vi "FrontPanel.vi"(8 "error in (no error)":errorcluster) -> (0 "error out":errorcluster)   [LabVIEW 2021]
uses:
  <vilib>/Native 3D Graph/xcontrol/3DPC_SurfacePlot.xctl
  QueueEnum.ctl
  ToViewQueueData.ctl
  ViewUpdateEnum.ctl
  ToControllerQueueCluster.ctl
  ToControllerEnum.ctl
panel:
  in  "Slide":dbl(slide) scale=0.0..100.0
  in  "See data from log file":bool
  in  "saving logs":bool
  in  "Log file":path
  in  "stop":bool
  in  "Send":bool
  in  "Message To Send":string
  out "3D Graph":refnum<class "Base Datatype.lvclass">[](xcontrol)
  out "Connected?":bool
  in  "Disconnect":bool
  in  "Connect":bool
  in  "Remote Port Number":u16
  in  "Server IP":string
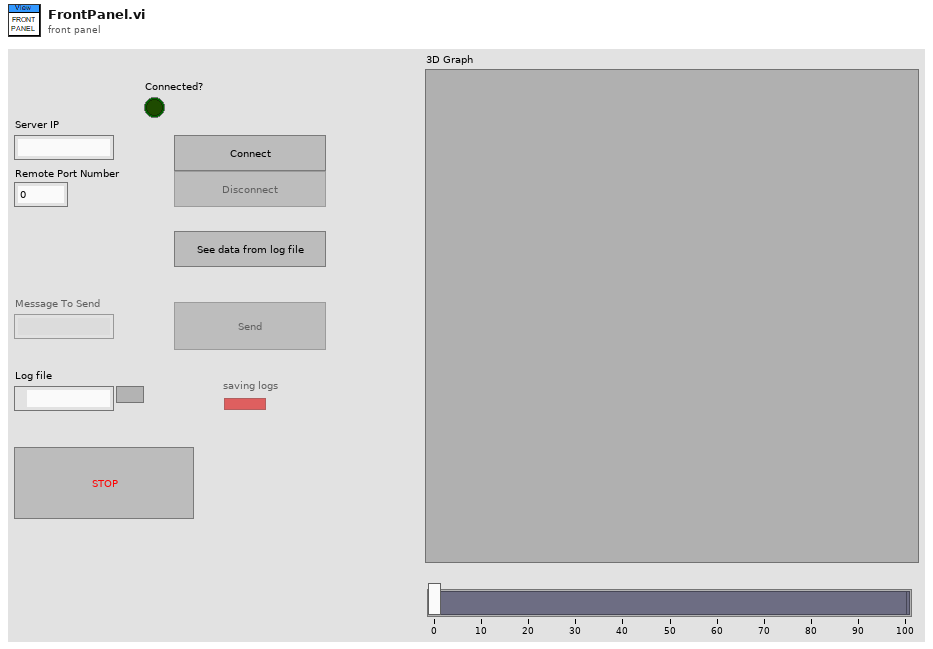
[diagram p1: front panel]
types:
  T1 = typedef "ToViewQueueData.ctl" = cluster{"DataToUpdate":T2, "ConnectionStatus":bool, "GraphData":dbl[][], "Message":string}
  T2 = typedef "ViewUpdateEnum.ctl" = enum16{"Init", "OneButtonMessage", "Exit", "UpdateButtonsEnabled", "UpdateGraph", "UpdateConnectionStatus"}
  T3 = enum32{"Bad", "Idle", "Run top level", "Running"}
  T4 = typedef "QueueEnum.ctl" = enum16{"Obtain Queue", "Get Queue Ref", "Flush Queue", "Release Queue"}
  T5 = typedef "ToControllerEnum.ctl" = enum16{"Info_Disconnected", "Info_Connected", "Exit", "Disconnect", "Connect", "SendMessage", "Slide", "ShowDataFromLog", "Start_Saving_Logs", "Stop_Saving_Logs"}
  T6 = typedef "ToControllerQueueCluster.ctl" = cluster{"Message":T5, "Remote IP":string, "Remote Port":u16, "Data":string}
  T7 = enum8{"Enabled", "Disabled", "Disabled and Grayed Out"}
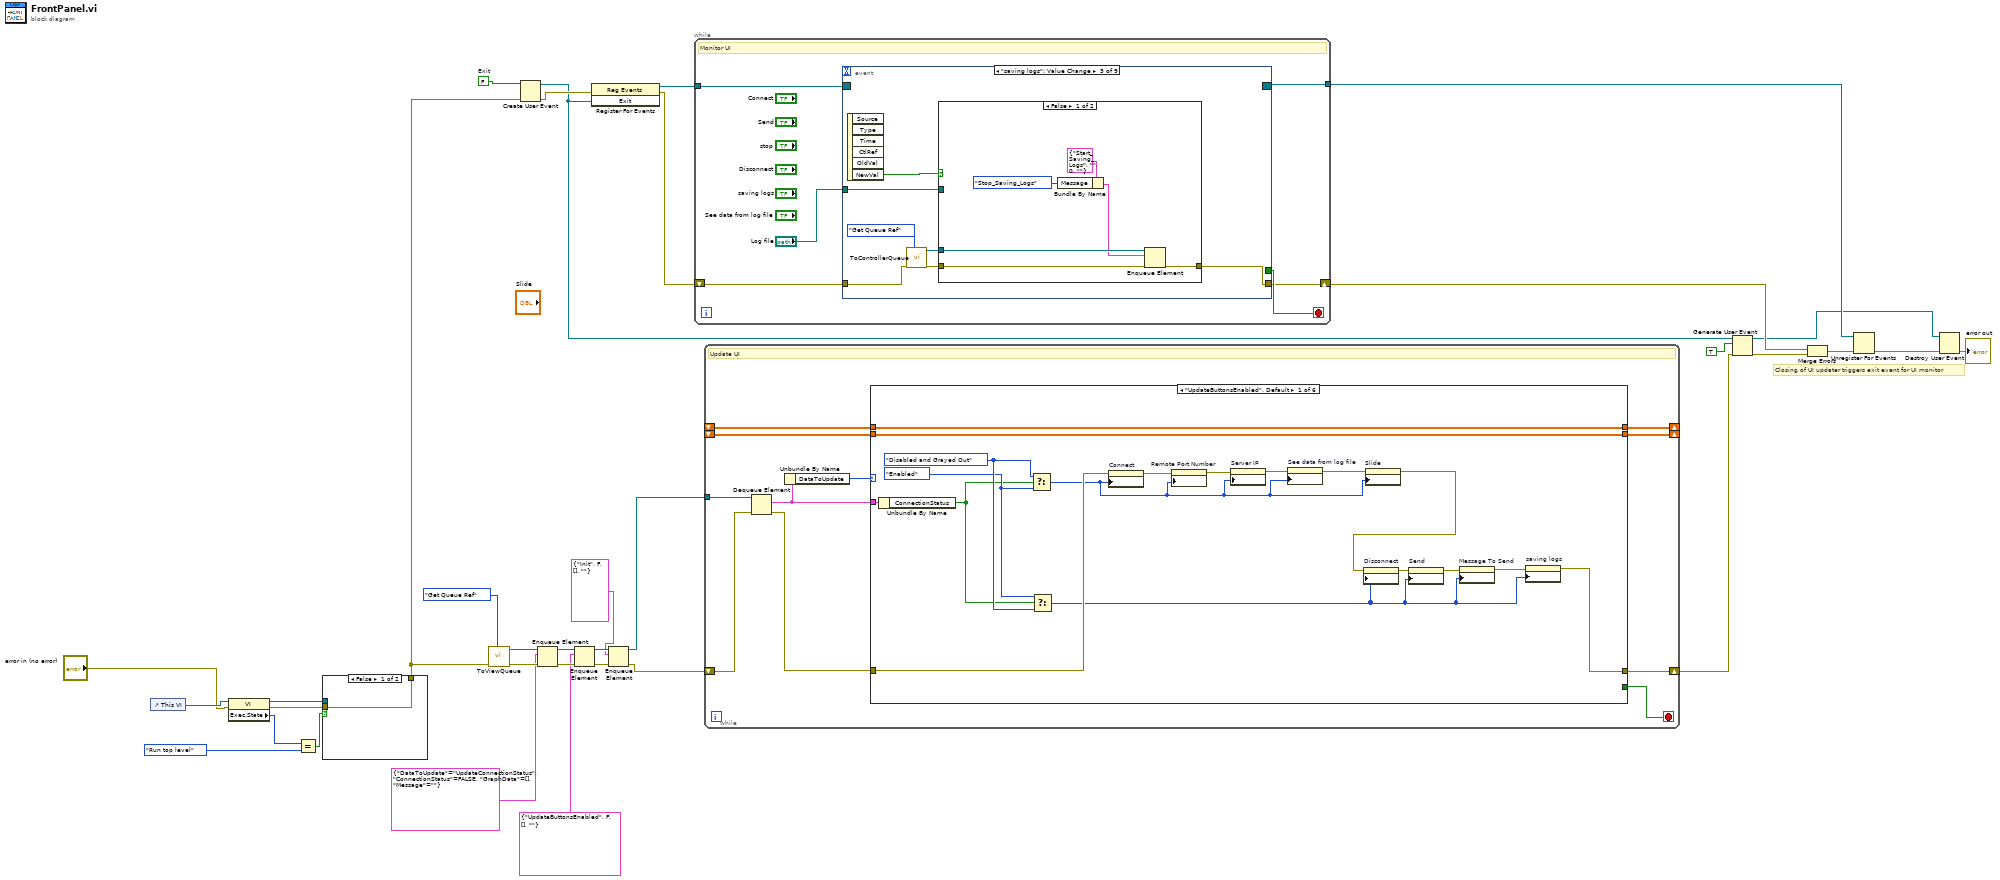
[diagram p0: block diagram]
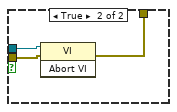
[diagram p2: hidden frame]
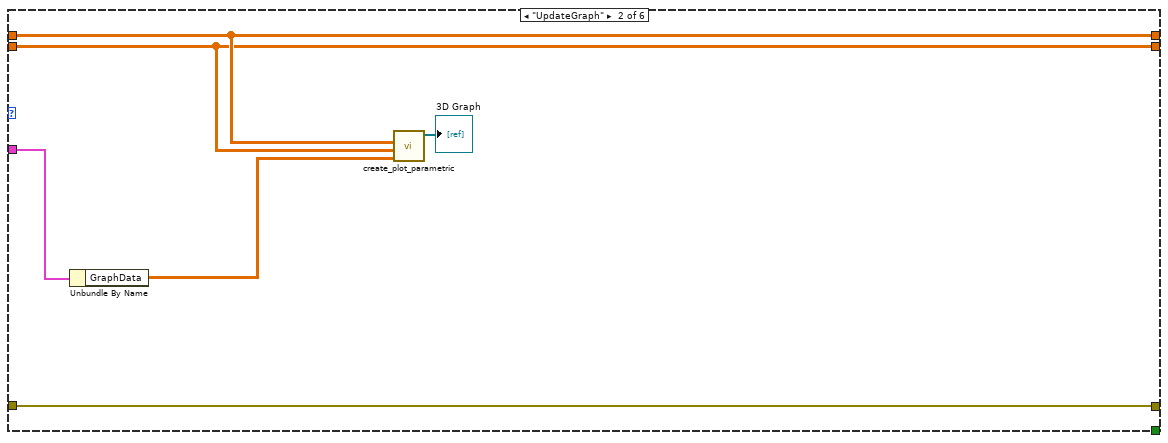
[diagram p3: hidden frame]
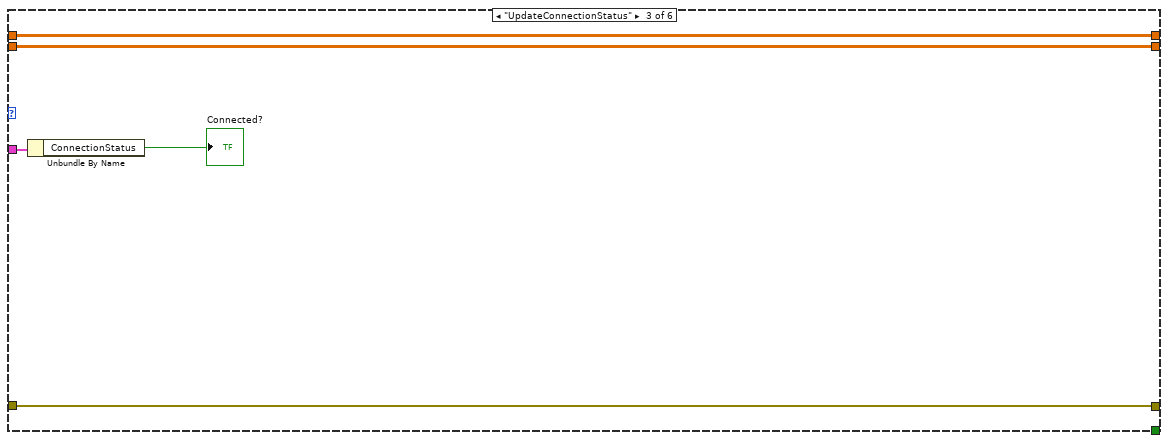
[diagram p4: hidden frame]
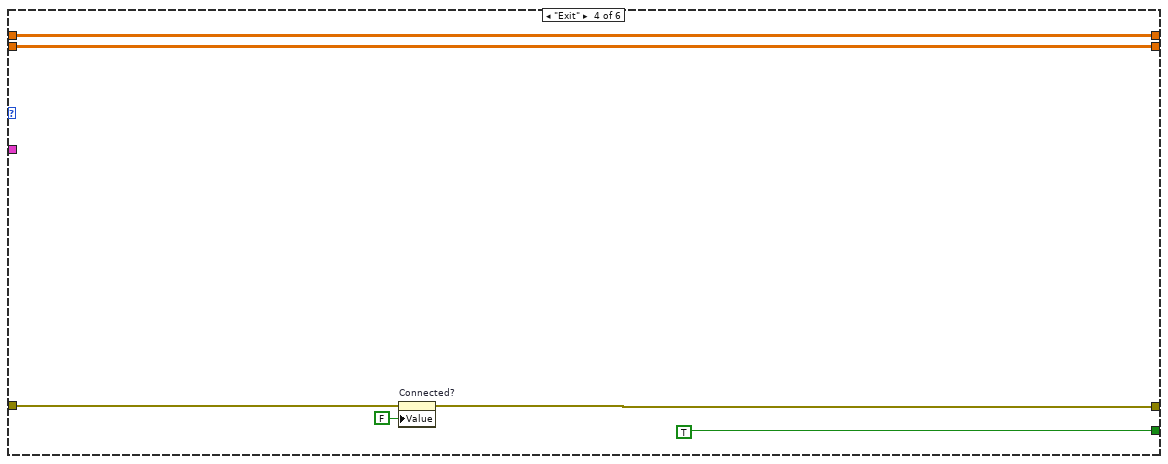
[diagram p5: hidden frame]
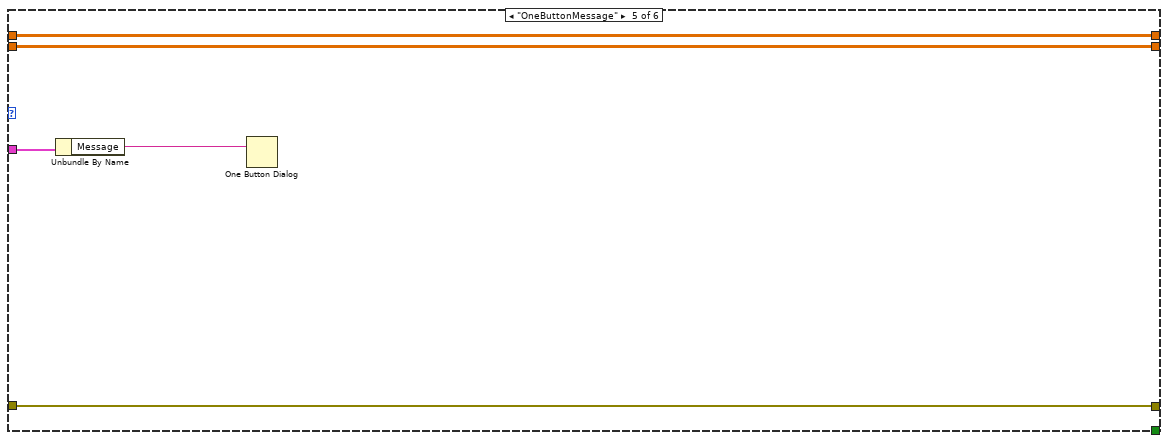
[diagram p6: hidden frame]
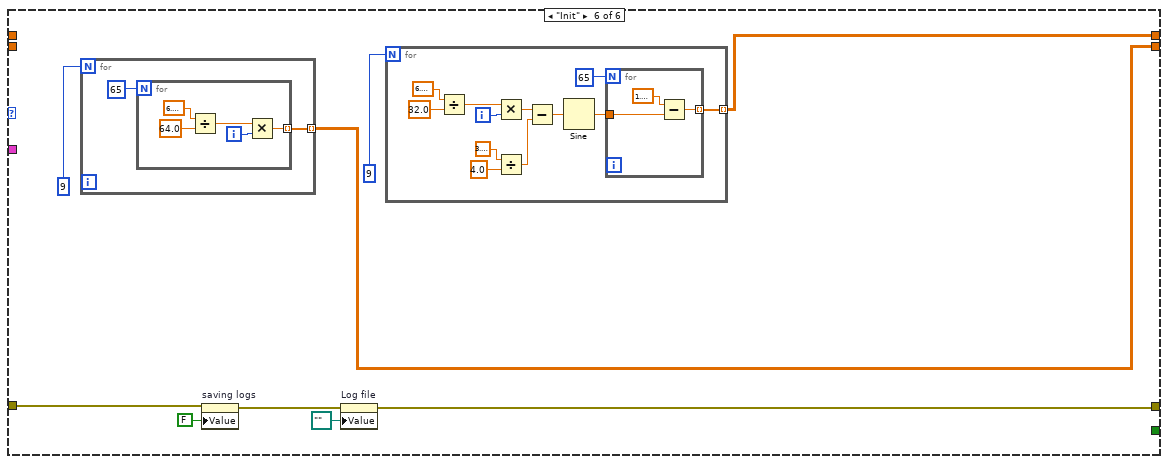
[diagram p7: hidden frame]
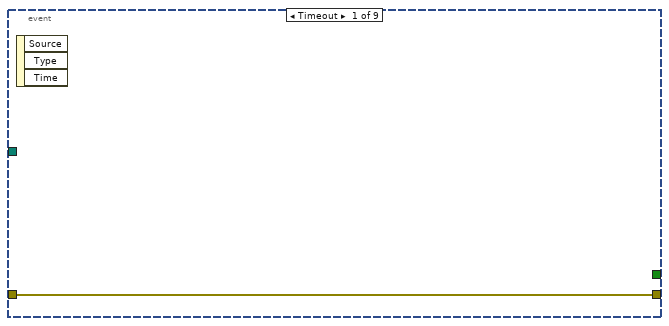
[diagram p8: hidden frame]
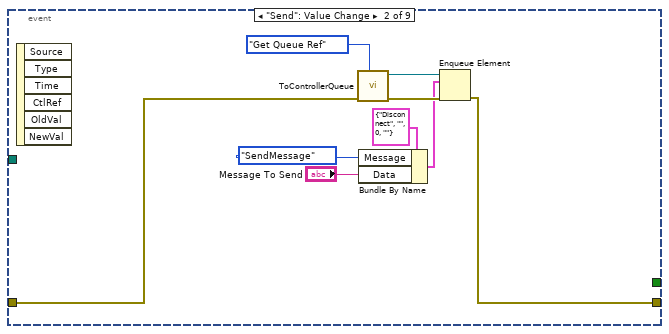
[diagram p9: hidden frame]
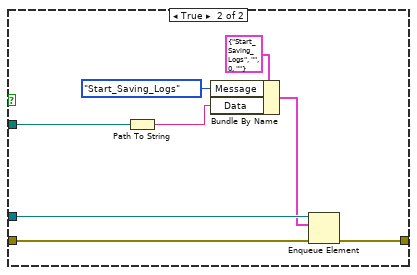
[diagram p10: hidden frame]
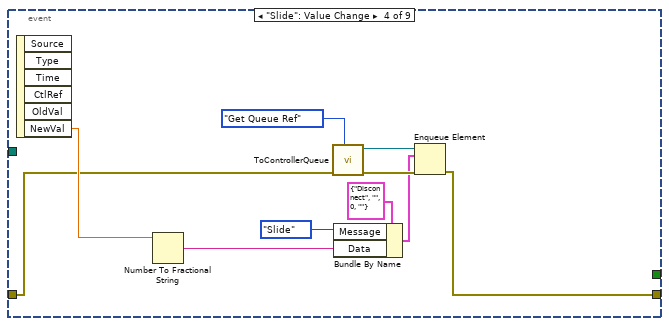
[diagram p11: hidden frame]
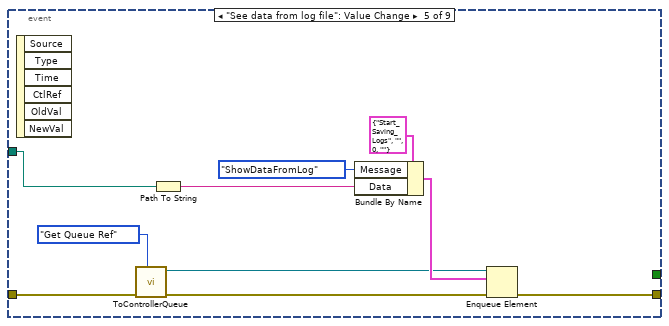
[diagram p12: hidden frame]
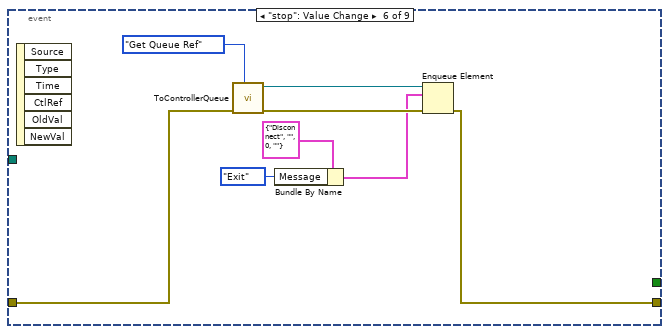
[diagram p13: hidden frame]
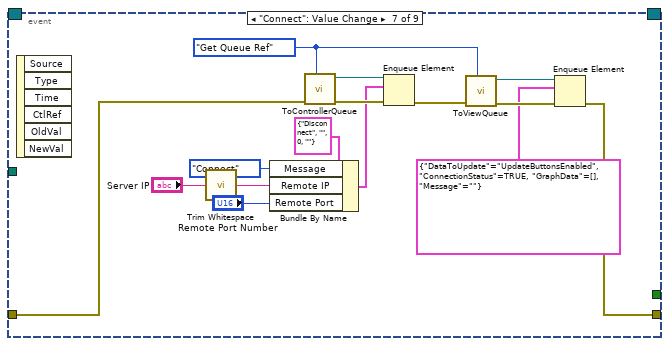
[diagram p14: hidden frame]
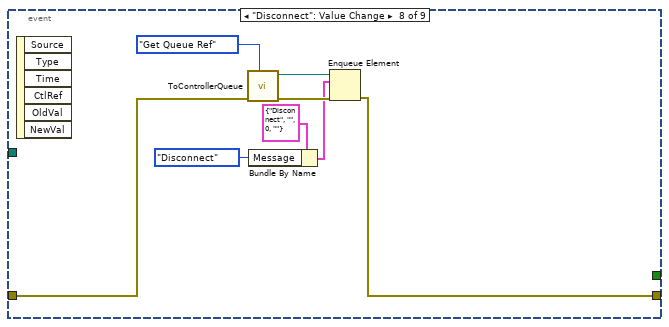
[diagram p15: hidden frame]
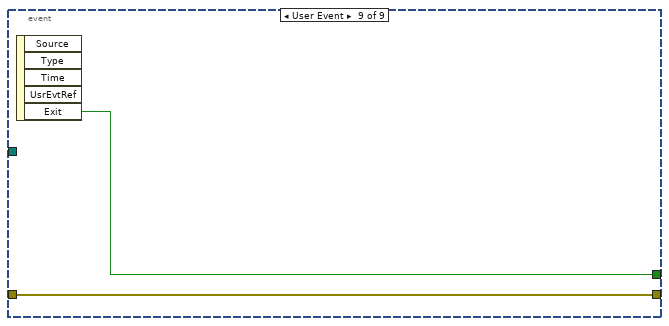
[diagram p16: hidden frame]
diagram:
  w33 = FALSE  # Exit
  # "Closing of UI updater triggers exit event for UI monitor"
  n1 = control-ref of="This VI"() -> (w17:refnum<vi>)
  n2 = property class="VI"(reference=w17, error in="error in (no error)") -> (reference out=w13:refnum<vi>, error out=w14:errorcluster, "Exec.State"=w15:T3)
  n3 = Equal?(x=w15, y=T3."Run top level" ("Execution:State")) -> (x = y?=w11:bool)
  n4 = case shown="False" w11 {
    tunnel: w14 -> [w35 w38]
    tunnel: w13 -> [_ w37]
    tunnel: [w35 w36] -> w21
    frame False {
    }
    frame True {
      n5 = invoke class="VI" method="Abort VI"(reference=w37, error in=w38) -> (error out=w36:errorcluster)  [unwired: 1 in, 2 out]
    }
  }
  n6 = call "ToViewQueue.vi"("Enum"=QueueEnum."Get Queue Ref", "error in (no error)"=w21) -> ("error out"=w9:errorcluster, "queue out"=w19:refnum<queue>)  [unwired: 8 in]
  n7 = Create User Event(user event datatype=w33, error in=w21) -> (user event=w23:refnum<user-event>, error out=w34:errorcluster)
  n8 = Enqueue Element(queue=w19, element=T1 {"DataToUpdate"=enum."UpdateConnectionStatus", "ConnectionStatus"=FALSE, "GraphData"=[], "Message"=""}, error in (no error)=w9) -> (queue out=w10:refnum<queue>, error out=w7:errorcluster)  [unwired: 1 in, 1 out]
  n9 = Enqueue Element(queue=w10, element=T1 {"DataToUpdate"=enum."UpdateButtonsEnabled", "ConnectionStatus"=FALSE, "GraphData"=[], "Message"=""}, error in (no error)=w7) -> (queue out=w8:refnum<queue>, error out=w3:errorcluster)  [unwired: 1 in, 1 out]
  n10 = register-events(error in=w34, w23) -> (reference out=w32:refnum<event-registration>, error out=w31:errorcluster)  [unwired: 1 in]
  n11 = Enqueue Element(queue=w8, element=T1 {"DataToUpdate"=enum."Init", "ConnectionStatus"=FALSE, "GraphData"=[], "Message"=""}, error in (no error)=w3) -> (queue out=w4:refnum<queue>, error out=w2:errorcluster)  [unwired: 1 in, 1 out]
  n12 = while {
    tunnel: w32 -> [w44]
    tunnel: [w41] -> w28
    shift-right: [w40] -> w26
    shift-left: w31 -> [w43]
    stop <- w42 stop-if-true
    # "Monitor UI"
    n13 = event shown="[2] \"saving logs\": Value Change" {
      selector: w44 -> [_ _ _ _ _ _ _ _ _]
      dyn-events: [_ _ _ _ _ _ _ _ _] -> w41
      timeout: _ -> [_ _ _ _ _ _ _ _ _]
      tunnel: w43 -> [w45 w48 w58 w77 w94 w102 w116 w119 w127]
      tunnel: [_ _ _ _ _ _ _ _ w128] -> w42
      tunnel: [w45 w47 w60 w76 w88 w100 w112 w120 w127] -> w40
      tunnel: "Log file" -> [_ _ w55 _ w87 _ _ _ _]
      event Timeout {
        n14 = event-data() -> ()  [unwired: 1 in, 3 out]
      }
      event "Send": Value Change {
        n15 = event-data() -> ()  [unwired: 1 in, 6 out]
        n16 = call "ToControllerQueue.vi"("Enum"=QueueEnum."Get Queue Ref", "error in (no error)"=w48) -> ("error out"=w54:errorcluster, "queue out"=w52:refnum<queue>)  [unwired: 8 in]
        n17 = Bundle By Name(cluster=T6 {"Message"=enum."Disconnect", "Remote IP"="", "Remote Port"=0, "Data"=""} ("element"), "Message"=ToControllerEnum."SendMessage", "Data"="Message To Send") -> (w49:T6)
        n18 = Enqueue Element(queue=w52, element=w49, error in (no error)=w54) -> (error out=w47:errorcluster)  [unwired: 1 in, 2 out]
      }
      event "saving logs": Value Change {
        n19 = event-data() -> ("NewVal"=w61:bool)  [unwired: 1 in, 5 out]
        n20 = call "ToControllerQueue.vi"("Enum"=QueueEnum."Get Queue Ref", "error in (no error)"=w58) -> ("error out"=w57:errorcluster, "queue out"=w56:refnum<queue>)  [unwired: 8 in]
        n21 = case shown="False" w61 {
          tunnel: w57 -> [w66 w75]
          tunnel: [w65 w73] -> w60
          tunnel: w56 -> [w67 w74]
          tunnel: w55 -> [_ w68]
          frame False {
            n22 = Bundle By Name(cluster=T6 {"Message"=enum."Start_Saving_Logs", "Remote IP"="", "Remote Port"=0, "Data"=""} ("element"), "Message"=ToControllerEnum."Stop_Saving_Logs") -> (w62:T6)
            n23 = Enqueue Element(queue=w67, element=w62, error in (no error)=w66) -> (error out=w65:errorcluster)  [unwired: 1 in, 2 out]
          }
          frame True {
            n24 = Path To String(path=w68) -> (string=w69:string)
            n25 = Bundle By Name(cluster=T6 {"Message"=enum."Start_Saving_Logs", "Remote IP"="", "Remote Port"=0, "Data"=""} ("element"), "Message"=ToControllerEnum."Start_Saving_Logs", "Data"=w69) -> (w71:T6)
            n26 = Enqueue Element(queue=w74, element=w71, error in (no error)=w75) -> (error out=w73:errorcluster)  [unwired: 1 in, 2 out]
          }
        }
      }
      event "Slide": Value Change {
        n27 = event-data() -> ("NewVal"=w78:dbl)  [unwired: 1 in, 5 out]
        n28 = Number To Fractional String(number=w78) -> (F-format string=w79:string)  [unwired: 3 in]
        n29 = call "ToControllerQueue.vi"("Enum"=QueueEnum."Get Queue Ref", "error in (no error)"=w77) -> ("error out"=w85:errorcluster, "queue out"=w83:refnum<queue>)  [unwired: 8 in]
        n30 = Bundle By Name(cluster=T6 {"Message"=enum."Disconnect", "Remote IP"="", "Remote Port"=0, "Data"=""} ("element"), "Message"=ToControllerEnum."Slide", "Data"=w79) -> (w80:T6)
        n31 = Enqueue Element(queue=w83, element=w80, error in (no error)=w85) -> (error out=w76:errorcluster)  [unwired: 1 in, 2 out]
      }
      event "See data from log file": Value Change {
        n32 = event-data() -> ()  [unwired: 1 in, 6 out]
        n33 = call "ToControllerQueue.vi"("Enum"=QueueEnum."Get Queue Ref", "error in (no error)"=w94) -> ("error out"=w89:errorcluster, "queue out"=w90:refnum<queue>)  [unwired: 8 in]
        n34 = Path To String(path=w87) -> (string=w86:string)
        n35 = Bundle By Name(cluster=T6 {"Message"=enum."Start_Saving_Logs", "Remote IP"="", "Remote Port"=0, "Data"=""} ("element"), "Message"=ToControllerEnum."ShowDataFromLog", "Data"=w86) -> (w91:T6)
        n36 = Enqueue Element(queue=w90, element=w91, error in (no error)=w89) -> (error out=w88:errorcluster)  [unwired: 1 in, 2 out]
      }
      event "stop": Value Change {
        n37 = event-data() -> ()  [unwired: 1 in, 6 out]
        n38 = call "ToControllerQueue.vi"("Enum"=QueueEnum."Get Queue Ref", "error in (no error)"=w102) -> ("error out"=w101:errorcluster, "queue out"=w99:refnum<queue>)  [unwired: 8 in]
        n39 = Bundle By Name(cluster=T6 {"Message"=enum."Disconnect", "Remote IP"="", "Remote Port"=0, "Data"=""} ("element"), "Message"=ToControllerEnum."Exit") -> (w96:T6)
        n40 = Enqueue Element(queue=w99, element=w96, error in (no error)=w101) -> (error out=w100:errorcluster)  [unwired: 1 in, 2 out]
      }
      event "Connect": Value Change {
        w114 = QueueEnum."Get Queue Ref"
        n41 = event-data() -> ()  [unwired: 1 in, 6 out]
        n42 = call <vilib>:"Trim Whitespace.vi"("string"="Server IP") -> ("trimmed string"=w104:string)  [unwired: 1 in]
        n43 = Bundle By Name(cluster=T6 {"Message"=enum."Disconnect", "Remote IP"="", "Remote Port"=0, "Data"=""} ("element"), "Message"=ToControllerEnum."Connect", "Remote IP"=w104, "Remote Port"="Remote Port Number") -> (w105:T6)
        n44 = call "ToControllerQueue.vi"("Enum"=w114, "error in (no error)"=w116) -> ("error out"=w118:errorcluster, "queue out"=w117:refnum<queue>)  [unwired: 8 in]
        n45 = Enqueue Element(queue=w117, element=w105, error in (no error)=w118) -> (error out=w115:errorcluster)  [unwired: 1 in, 2 out]
        n46 = call "ToViewQueue.vi"("Enum"=w114, "error in (no error)"=w115) -> ("error out"=w113:errorcluster, "queue out"=w111:refnum<queue>)  [unwired: 8 in]
        n47 = Enqueue Element(queue=w111, element=T1 {"DataToUpdate"=enum."UpdateButtonsEnabled", "ConnectionStatus"=TRUE, "GraphData"=[], "Message"=""} ("ViewQueueData"), error in (no error)=w113) -> (error out=w112:errorcluster)  [unwired: 1 in, 2 out]
      }
      event "Disconnect": Value Change {
        n48 = event-data() -> ()  [unwired: 1 in, 6 out]
        n49 = call "ToControllerQueue.vi"("Enum"=QueueEnum."Get Queue Ref", "error in (no error)"=w119) -> ("error out"=w126:errorcluster, "queue out"=w124:refnum<queue>)  [unwired: 8 in]
        n50 = Bundle By Name(cluster=T6 {"Message"=enum."Disconnect", "Remote IP"="", "Remote Port"=0, "Data"=""} ("element"), "Message"=ToControllerEnum."Disconnect") -> (w121:T6)
        n51 = Enqueue Element(queue=w124, element=w121, error in (no error)=w126) -> (error out=w120:errorcluster)  [unwired: 1 in, 2 out]
      }
      event User Event {
        n52 = event-data() -> ("Exit"=w128:bool)  [unwired: 1 in, 4 out]
      }
    }
  }
  n53 = while {
    shift-right: [w134] -> w30
    shift-left: w2 -> [w138]
    tunnel: w4 -> [w139]
    shift-right: [w130] -> _
    shift-left: _ -> [w131]
    shift-right: [w129] -> _
    shift-left: _ -> [w132]
    stop <- w133 stop-if-true
    # "Update UI"
    n54 = Dequeue Element(queue=w139, error in (no error)=w138) -> (element=w135:T1, error out=w137:errorcluster)  [unwired: 1 in, 2 out]
    n55 = Unbundle By Name(w135) -> ("DataToUpdate"=w136:T2)
    n56 = case shown="\"UpdateButtonsEnabled\", Default" w136 {
      tunnel: w137 -> [w152 w163 w168 w173 w177 w184]
      tunnel: w135 -> [w157 w161 w167 _ w179 _]
      tunnel: [w144 w163 w168 w172 w177 w182] -> w134
      tunnel: [_ _ _ TRUE _ _] -> w133
      tunnel: w132 -> [w148 w160 w164 w169 w175 _]
      tunnel: w131 -> [w149 w159 w165 w170 w176 _]
      tunnel: [w149 w159 w165 w170 w176 w186] -> w130
      tunnel: [w148 w160 w164 w169 w175 w185] -> w129
      frame "UpdateButtonsEnabled", Default {
        w153 = T7."Enabled" ("Disabled")
        w154 = T7."Disabled and Grayed Out" ("Disabled")
        n57 = Unbundle By Name(w157) -> ("ConnectionStatus"=w146:bool)
        n58 = Select(t=w154, s=w146, f=w153) -> (s? t:f=w141:T7)
        n59 = Select(t=w153, s=w146, f=w154) -> (s? t:f=w145:T7)
        n60 = property on="Connect" class="Bool"(error in=w152, "DisabledEnum"=w141) -> (error out=w156:errorcluster)  [unwired: 1 in, 1 out]
        n61 = property on="Remote Port Number" class="DigNum (strict)"(error in=w156, "DisabledEnum"=w141) -> (error out=w155:errorcluster)  [unwired: 1 in, 1 out]
        n62 = property on="Server IP" class="Str"(error in=w155, "DisabledEnum"=w141) -> (error out=w143:errorcluster)  [unwired: 1 in, 1 out]
        n63 = property on="See data from log file" class="Bool"(error in=w143, "DisabledEnum"=w141) -> (error out=w142:errorcluster)  [unwired: 1 in, 1 out]
        n64 = property on="Slide" class="Slide (strict)"(error in=w142, "DisabledEnum"=w141) -> (error out=w140:errorcluster)  [unwired: 1 in, 1 out]
        n65 = property on="Disconnect" class="Bool"(error in=w140, "DisabledEnum"=w145) -> (error out=w151:errorcluster)  [unwired: 1 in, 1 out]
        n66 = property on="Send" class="Bool"(error in=w151, "DisabledEnum"=w145) -> (error out=w150:errorcluster)  [unwired: 1 in, 1 out]
        n67 = property on="Message To Send" class="Str"(error in=w150, "DisabledEnum"=w145) -> (error out=w147:errorcluster)  [unwired: 1 in, 1 out]
        n68 = property on="saving logs" class="Bool (strict)"(error in=w147, "DisabledEnum"=w145) -> (error out=w144:errorcluster)  [unwired: 1 in, 1 out]
      }
      frame "UpdateGraph" {
        n69 = Unbundle By Name(w161) -> ("GraphData"=w158:dbl[][])
        n70 = call <vilib>:"create_plot_parametric.vi"("z matrix"=w158, "y matrix"=w159, "x matrix"=w160) -> ("plots out"=→"3D Graph":refnum<class "Base Datatype.lvclass">[])  [unwired: 2 in, 6 out]
      }
      frame "UpdateConnectionStatus" {
        n71 = Unbundle By Name(w167) -> ("ConnectionStatus"=→"Connected?":bool)
      }
      frame "Exit" {
        n72 = property on="Connected?" class="Bool (strict)"(error in=w173, "Value"=FALSE ("Connected?")) -> (error out=w172:errorcluster)  [unwired: 1 in, 1 out]
      }
      frame "OneButtonMessage" {
        n73 = Unbundle By Name(w179) -> ("Message"=w178:string)
        n74 = One Button Dialog(message=w178) -> ()  [unwired: 1 in, 1 out]
      }
      frame "Init" {
        n75 = for {
          N: 9 -> [_]
          tunnel: [w189] -> w186 mode=indexing
          n76 = for {
            N: 65 -> [_]
            tunnel: [w192] -> w189 mode=indexing
            i -> [w193]
            n77 = Divide(x=6.283185307179586, y=64.0) -> (x/y=w194:dbl)
            n78 = Multiply(x=w194, y=w193) -> (x*y=w192:dbl)
          }
        }
        n79 = property on="saving logs" class="Bool (strict)"(error in=w184, "Value"=FALSE ("save logs")) -> (error out=w183:errorcluster)  [unwired: 1 in, 1 out]
        n80 = property on="Log file" class="Path"(error in=w183, "Value"=path "" ("Log file")) -> (error out=w182:errorcluster)  [unwired: 1 in, 1 out]
        n81 = for {
          N: 9 -> [_]
          tunnel: [w197] -> w185 mode=indexing
          i -> [w205]
          n82 = Divide(x=6.283185307179586, y=32.0) -> (x/y=w206:dbl)
          n83 = Multiply(x=w206, y=w205) -> (x*y=w202:dbl)
          n84 = Divide(x=3.141592653589793, y=4.0) -> (x/y=w199:dbl)
          n85 = Subtract(x=w202, y=w199) -> (x-y=w203:dbl)
          n86 = Sine(x=w203) -> (sin(x)=w198:dbl)
          n87 = for {
            N: 65 -> [_]
            tunnel: w198 -> [w209]
            tunnel: [w208] -> w197 mode=indexing
            n88 = Subtract(x=1.5707963267948966, y=w209) -> (x-y=w208:dbl)
          }
        }
      }
    }
  }
  n89 = Generate User Event(user event=w23, event data cluster=TRUE ("event data"), error in=w30) -> (user event out=w22:refnum<user-event>, error out=w27:errorcluster)  [unwired: 1 in]
  n90 = Merge Errors(w26, w27) -> (w25:errorcluster)
  n91 = Unregister For Events(event registration refnum=w28, error in=w25) -> (error out=w24:errorcluster)
  n92 = Destroy User Event(user event=w22, error in=w24) -> (error out=→"error out":errorcluster)
